vi "Typecast.vi"(8 "error in (no error)":errorcluster, 11 "Decode_Packet in":refnum<class "Decode_Packet.lvclass">) -> (0 "error out":errorcluster, 3 "Pupil_Diameter out":refnum<class "Gaze.lvclass">)   [LabVIEW 2020, in "Gaze.lvclass"]
uses:
  Gaze.lvclass
  Decode_Packet/Decode_Packet.lvclass
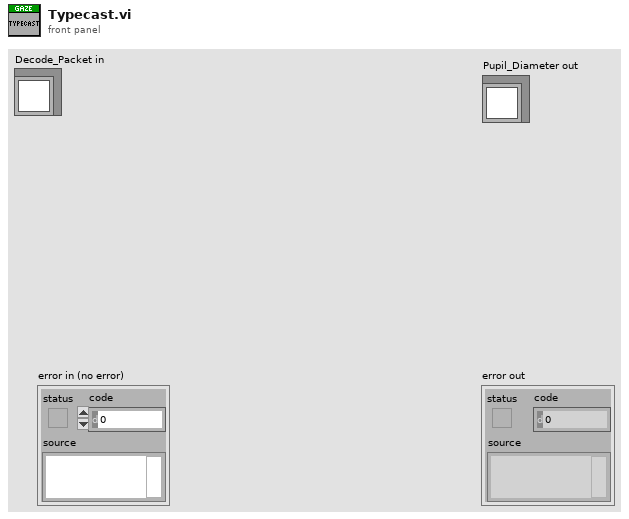
[diagram p1: front panel]
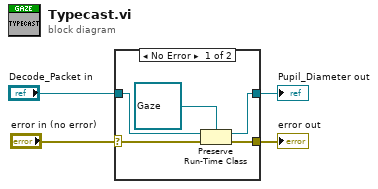
[diagram p0: block diagram]
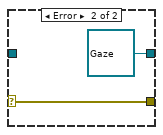
[diagram p2: hidden frame]
diagram:
  n1 = case shown="No Error" "error in (no error)" {
    selector: "error in (no error)" -> [w9 w11]
    tunnel: [w8 w11] -> w3
    tunnel: [w7 refnum<class "Gaze.lvclass"> refnum ("Pupil_Diameter in")] -> w2
    tunnel: "Decode_Packet in" -> [w5 _]
    frame No Error {
      n2 = Preserve Run-Time Class(object in=w5, error in=w9, 2:refnum<class "Gaze.lvclass"> refnum ("Pupil_Diameter in")) -> (object out=w7:refnum<class "Gaze.lvclass">, error out=w8:errorcluster)
    }
    frame Error {
    }
  }
  "error out" <- w3
  "Pupil_Diameter out" <- w2
